vi "Parse Domain Name.vi"(10 "offset":u16, 11 "message":string) -> (2 "offset past domain name":u16, 3 "domain name":string)   [LabVIEW 2015, in "PL DNS Client.lvlib"]
doc: "Parses domain name at specific <b>offset</b> in DNS <b>message</b>."
uses:
  PL DNS Client.lvlib
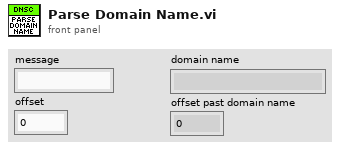
[diagram p1: front panel]
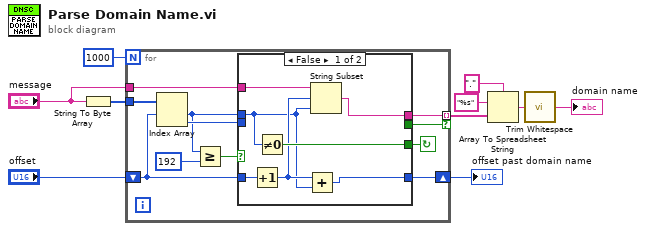
[diagram p0: block diagram]
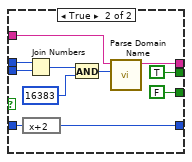
[diagram p2: hidden frame]
diagram:
  n1 = String To Byte Array(string="message") -> (unsigned byte array=w2:u8[])
  n2 = for {
    N: 1000 -> [_]
    tunnel: [w21] -> w5 mode=indexing if=w14
    shift-right: [w15] -> w3
    shift-left: "offset" -> [w16]
    tunnel: w2 -> [w13]
    tunnel: "message" -> [w11]
    stop <- w12 continue-if-true
    n3 = Index Array(array=w13, index #1=w16) -> (element #1=w17:u8, element #2=w18:u8)  [unwired: 1 in]
    n4 = Greater Or Equal?(x=w17, y=u8 192) -> (x >= y?=w19:bool)
    n5 = case shown="False" w19 {
      tunnel: [w24 w32] -> w21
      tunnel: [w25 TRUE] -> w14
      tunnel: w18 -> [_ w36]
      tunnel: w17 -> [w22 w37]
      tunnel: w16 -> [w27 w39]
      tunnel: [w26 w38] -> w15
      tunnel: w11 -> [w28 w31]
      tunnel: [w25 FALSE] -> w12
      frame False {
        n6 = Increment(x=w27) -> (x+1=w23:u16)
        n7 = Not Equal To 0?(x=w22) -> (x != 0?=w25:bool)
        n8 = Add(x=w23, y=w22) -> (x+y=w26:u16)
        n9 = String Subset(string=w28, offset (0)=w23, length (rest)=w22) -> (substring=w24:string)
      }
      frame True {
        n10 = expression code="x+2"(w39) -> (w38:u16)
        n11 = Join Numbers(hi=w37, lo=w36) -> ((hi.lo)=w34:u16)
        n12 = And(x=w34, y=u16 16383) -> (x .and. y?=w33:u16)
        n13 = call "Parse Domain Name.vi"("offset"=w33, "message"=w31) -> ("domain name"=w32:string)  [unwired: 8 in, 1 out]
      }
    }
  }
  "offset past domain name" <- w3
  n14 = Array To Spreadsheet String(delimiter (Tab)=".", array=w5, 3:"%s" ("format string")) -> (spreadsheet string=w7:string)
  n15 = call <vilib>:"Trim Whitespace.vi"("string"=w7) -> ("trimmed string"=→"domain name":string)  [unwired: 1 in]
